vi "告警参数.vi"() -> ()   [LabVIEW 2016, in "斯坦道CODMn.lvlib"]
uses:
  <vilib>/Plasmionique/MB Master/MB Master.lvlib
panel:
  in  "告警参数":T1={"F0阈值"=3000, "F1阈值"=3000, "F2阈值"=850, "F3-F2阈值"=50, "F4阈值 "=3000, "F4-F3阈值"=15, "F5阈值"=3000, "F5上限"=4000}
  in  "读取":bool
  in  "写入":bool
  in  "关闭":bool
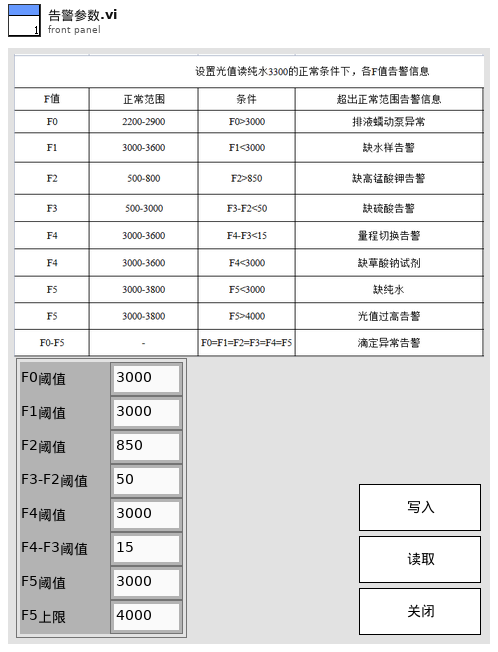
[diagram p1: front panel]
types:
  T1 = cluster{"F0阈值":u16, "F1阈值":u16, "F2阈值":u16, "F3-F2阈值":u16, "F4阈值 ":u16, "F4-F3阈值":u16, "F5阈值":u16, "F5上限":u16}
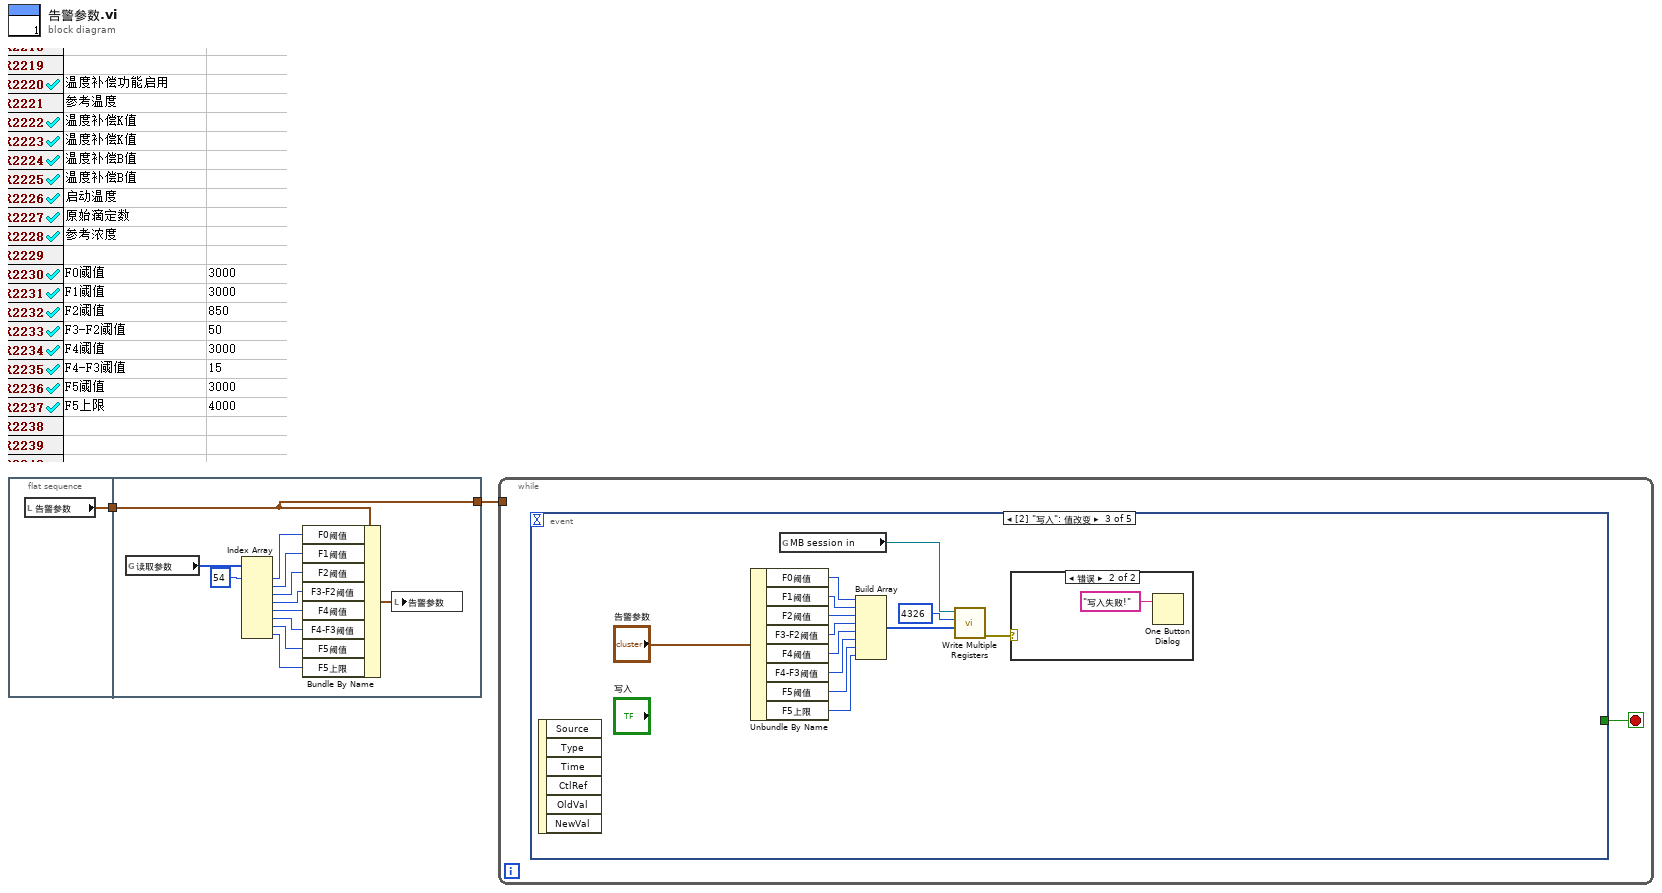
[diagram p0: block diagram]
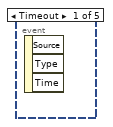
[diagram p2: hidden frame]
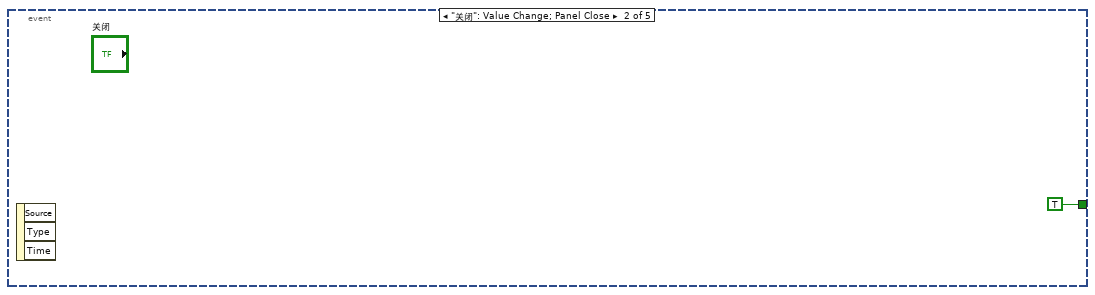
[diagram p3: hidden frame]
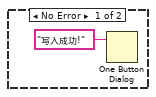
[diagram p4: hidden frame]
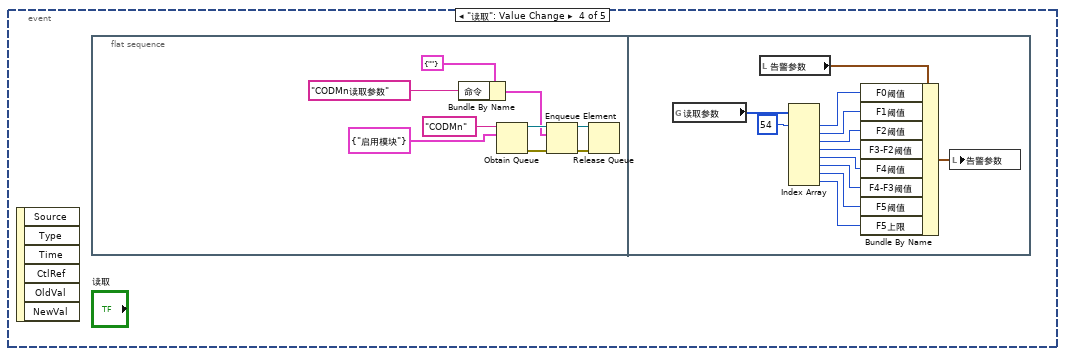
[diagram p5: hidden frame]
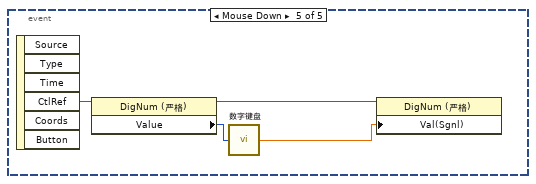
[diagram p6: hidden frame]
diagram:
  n1 = flat-sequence {
    tunnel: [w3] -> w1
    tunnel: [w4] -> w2
    tunnel: w1 -> [w4]
    frame #0 {
      n2 = local read "告警参数"() -> (w3:T1)
    }
    frame #1 {
      n3 = global read "COD内部交互全局.vi" "读取参数"() -> (w7:u16[])
      n4 = Index Array(array=w7, index #1=54 ("索引")) -> (element #1=w8:u16, element #2=w9:u16, element #3=w10:u16, element #4=w11:u16, element #5=w12:u16, element #6=w13:u16, element #7=w14:u16, element #8=w15:u16)  [unwired: 7 in]
      n5 = Bundle By Name(cluster=w4, "F0阈值"=w8, "F1阈值"=w9, "F2阈值"=w10, "F3-F2阈值"=w11, "F4阈值"=w12, "F4-F3阈值"=w13, "F5阈值"=w14, "F5上限"=w15) -> (w5:T1)
      n6 = local write "告警参数"(w5) -> ()
    }
  }
  n7 = while {
    tunnel: w2 -> [_]
    stop <- w16 stop-if-true
    n8 = event shown="[2] \"写入\": 值改变" {
      selector: _ -> [_ _ _ _ _]
      dyn-events: _ -> [_ _ _ _ _]
      timeout: _ -> [_ _ _ _ _]
      tunnel: [_ TRUE _ _ _] -> w16
      event Timeout {
        n9 = event-data() -> ()  [unwired: 1 in, 3 out]
      }
      event "关闭": Value Change; Panel Close {
        n10 = event-data() -> ()  [unwired: 1 in, 3 out]
      }
      event "写入": Value Change {
        n11 = event-data() -> ()  [unwired: 1 in, 6 out]
        n12 = Unbundle By Name("告警参数") -> ("F0阈值"=w27:u16, "F1阈值"=w26:u16, "F2阈值"=w25:u16, "F3-F2阈值"=w24:u16, "F4阈值"=w23:u16, "F4-F3阈值"=w22:u16, "F5阈值"=w21:u16, "F5上限"=w20:u16)
        n13 = global read "COD浓度全局变量.vi" "MB session in"() -> (w30:refnum<class "MB_Master.lvclass">)
        n14 = Build Array(w27, w26, w25, w24, w23, w22, w21, w20) -> (w19:u16[])
        n15 = call <vilib>:"Write Multiple Registers.vi"("values"=w19, "starting address"=u16 4326, "MB session in"=w30) -> ("error out"=w18:errorcluster)  [unwired: 7 in, 1 out]
        n16 = case shown="错误" w18 {
          frame No Error {
            n17 = One Button Dialog(message="写入成功!" ("消息")) -> ()  [unwired: 1 in, 1 out]
          }
          frame Error {
            n18 = One Button Dialog(message="写入失败!" ("消息")) -> ()  [unwired: 1 in, 1 out]
          }
        }
      }
      event "读取": Value Change {
        n19 = event-data() -> ()  [unwired: 1 in, 6 out]
        n20 = flat-sequence {
          frame #0 {
            n21 = Bundle By Name(cluster=cluster{"命令":string} {"命令"=""} ("元素"), "命令"="CODMn读取参数" ("名称（未命名）")) -> (w35:cluster{"命令":string})
            n22 = Obtain Queue(name (unnamed)="CODMn", element data type=cluster{"命令":string} {"命令"="启用模块"} ("元素")) -> (queue out=w40:refnum<queue>, error out=w41:errorcluster)  [unwired: 3 in, 1 out]
            n23 = Enqueue Element(queue=w40, element=w35, error in (no error)=w41) -> (queue out=w38:refnum<queue>, error out=w39:errorcluster)  [unwired: 1 in, 1 out]
            n24 = Release Queue(queue=w38, error in (no error)=w39) -> ()  [unwired: 1 in, 3 out]
          }
          frame #1 {
            n25 = global read "COD内部交互全局.vi" "读取参数"() -> (w52:u16[])
            n26 = local read "告警参数"() -> (w51:T1)
            n27 = Index Array(array=w52, index #1=54 ("索引")) -> (element #1=w49:u16, element #2=w48:u16, element #3=w47:u16, element #4=w46:u16, element #5=w45:u16, element #6=w44:u16, element #7=w43:u16, element #8=w42:u16)  [unwired: 7 in]
            n28 = Bundle By Name(cluster=w51, "F0阈值"=w49, "F1阈值"=w48, "F2阈值"=w47, "F3-F2阈值"=w46, "F4阈值"=w45, "F4-F3阈值"=w44, "F5阈值"=w43, "F5上限"=w42) -> (w50:T1)
            n29 = local write "告警参数"(w50) -> ()
          }
        }
      }
      event "告警参数.F0阈值", "告警参数.F1阈值", "告警参数.F2阈值", "告警参数.F3-F2阈值", "告警参数.F4阈值", "告警参数.F4-F3阈值", "告警参数.F5阈值", "告警参数.F5上限": Mouse Down {
        n30 = event-data() -> ("CtlRef"=w57:refnum<vi>)  [unwired: 1 in, 5 out]
        n31 = property class="DigNum (严格)"(reference=w57) -> (reference out=w55:refnum<vi>, "Value"=w56:u16)  [unwired: 1 in, 1 out]
        n32 = call "数字键盘.vi"("OldNumber"=w56) -> ("NewNumber"=w54:sgl)
        n33 = property class="DigNum (严格)"(reference=w55, "Val(Sgnl)"=w54) -> ()  [unwired: 1 in, 2 out]
      }
    }
  }
